vi "Auto_Routine_UTurnBalance.vi"(8 "error in (no error)":errorcluster, 11 "IsBlue?":bool) -> (0 "error out":errorcluster)   [LabVIEW 2020]
doc: "Drives a U Turn than balances. Determines if alliance is blue or red and adjusts accordingly.\n\ninputs:\n--IsBlue?--Boolean--\n--ErrorIn--\noutputs:\n--ErrorOut--"
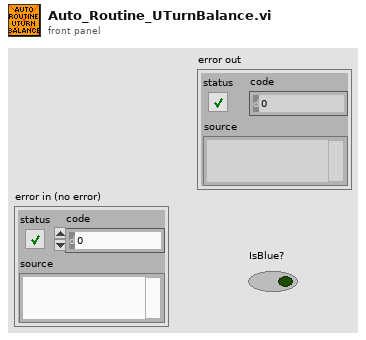
[diagram p1: front panel]
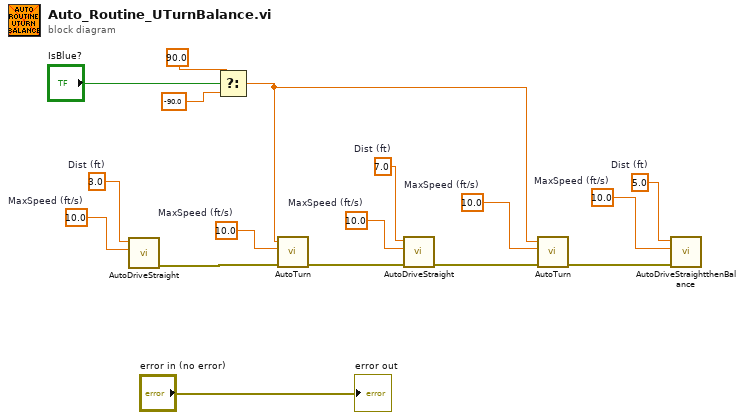
[diagram p0: block diagram]
diagram:
  w5 = 5.0  # Dist (ft)
  w6 = 10.0  # MaxSpeed (ft/s)
  w9 = 10.0  # MaxSpeed (ft/s)
  w11 = 10.0  # MaxSpeed (ft/s)
  w12 = 7.0  # Dist (ft)
  w14 = 10.0  # MaxSpeed (ft/s)
  w15 = 10.0  # MaxSpeed (ft/s)
  w16 = 3.0  # Dist (ft)
  n1 = call "AutoDriveStraight.vi"("MaxSpeed (ft/s)"=w15, "Dist (ft)"=w16) -> ("error out"=w13:errorcluster)  [unwired: 9 in]
  n2 = Select(t=90.0, s="IsBlue?", f=-90.0) -> (s? t:f=w1:dbl)
  n3 = call "AutoTurn.vi"("error in (no error)"=w13, "MaxSpeed (ft/s)"=w14, "degrees"=w1) -> ("error out"=w10:errorcluster)  [unwired: 8 in]
  n4 = call "AutoDriveStraight.vi"("error in (no error)"=w10, "MaxSpeed (ft/s)"=w11, "Dist (ft)"=w12) -> ("error out"=w8:errorcluster)  [unwired: 8 in]
  n5 = call "AutoTurn.vi"("error in (no error)"=w8, "MaxSpeed (ft/s)"=w9, "degrees"=w1) -> ("error out"=w7:errorcluster)  [unwired: 8 in]
  n6 = call "AutoDriveStraightthenBalance.vi"("error in (no error)"=w7, "MaxSpeed (ft/s)"=w6, "Dist (ft)"=w5) -> ()  [unwired: 8 in, 1 out]
  "error out" <- "error in (no error)"
